vi "Inpterpolate8.vi"(0 "X":fxp<+/-,16,14>, 11 "input valid":bool=TRUE) -> (2 "X(t -7)":fxp<+/-,16,14>, 3 "X(t -5)":fxp<+/-,16,14>, 4 "X(t)":fxp<+/-,16,14>, 6 "X(t -1)":fxp<+/-,16,14>, 8 "X(t -2)":fxp<+/-,16,14>, 10 "X(t -3)":fxp<+/-,16,14>, 13 "X(t -6)":fxp<+/-,16,14>, 14 "X(t -4)":fxp<+/-,16,14>, 15 "output valid":bool)   [LabVIEW 2013]
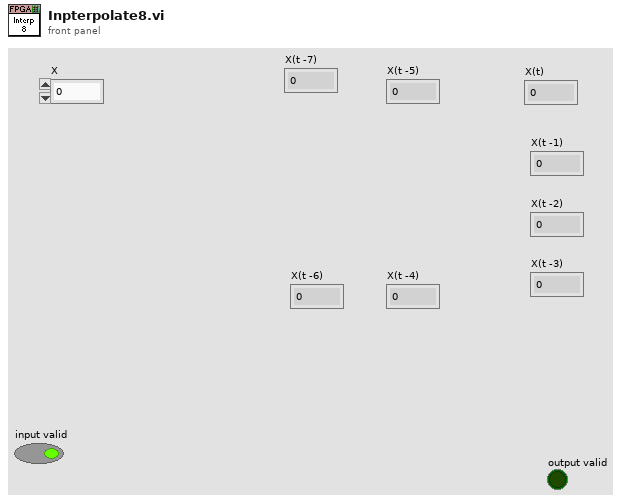
[diagram p1: front panel]
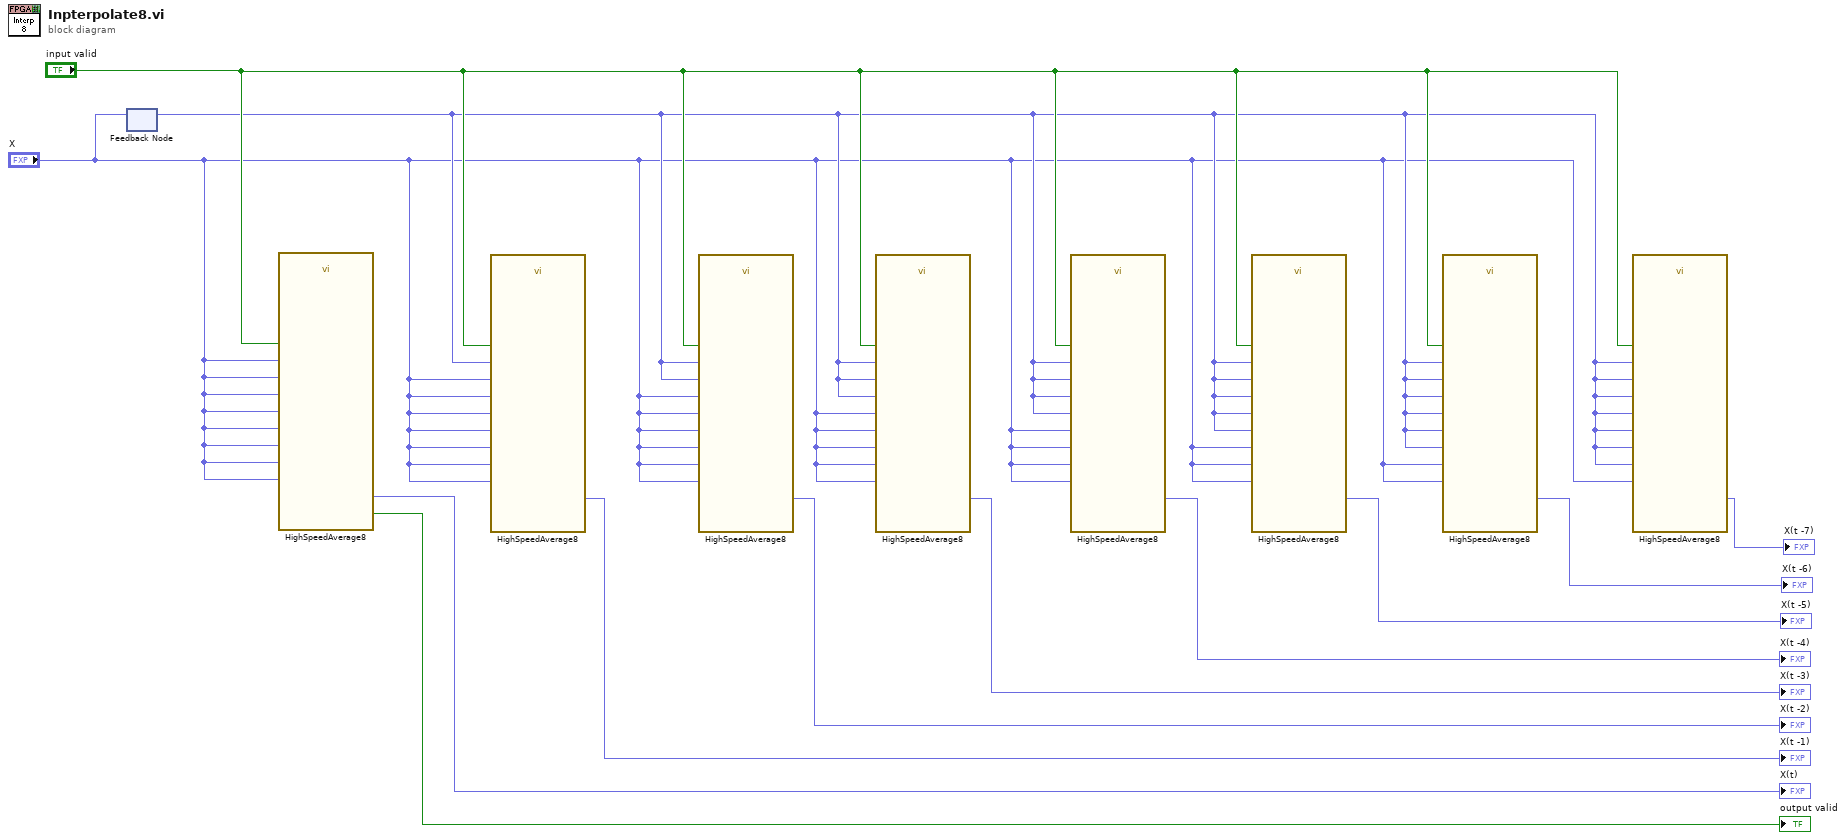
[diagram p0: block diagram]
diagram:
  n1 = feedback #1() -> (w2:fxp<+/-,16,14>)  [unwired: 1 in]
  n2 = feedback-in #1("X") -> ()
  n3 = call "HighSpeedAverage8.vi"("x 1"="X", "x 5"="X", "x 6"="X", "x 2"="X", "x 3"="X", "x 4"="X", "input valid"="input valid", "x 7"="X", "x 8"="X") -> ("average"=→"X(t)":fxp<+/-,16,14>, "output valid"=→"output valid":bool)  [unwired: 5 in]
  n4 = call "HighSpeedAverage8.vi"("x 1"=w2, "x 5"="X", "x 6"="X", "x 2"="X", "x 3"="X", "x 4"="X", "input valid"="input valid", "x 7"="X", "x 8"="X") -> ("average"=→"X(t -1)":fxp<+/-,16,14>)  [unwired: 5 in, 1 out]
  n5 = call "HighSpeedAverage8.vi"("x 1"=w2, "x 5"="X", "x 6"="X", "x 2"=w2, "x 3"="X", "x 4"="X", "input valid"="input valid", "x 7"="X", "x 8"="X") -> ("average"=→"X(t -2)":fxp<+/-,16,14>)  [unwired: 5 in, 1 out]
  n6 = call "HighSpeedAverage8.vi"("x 1"=w2, "x 5"="X", "x 6"="X", "x 2"=w2, "x 3"=w2, "x 4"="X", "input valid"="input valid", "x 7"="X", "x 8"="X") -> ("average"=→"X(t -3)":fxp<+/-,16,14>)  [unwired: 5 in, 1 out]
  n7 = call "HighSpeedAverage8.vi"("x 1"=w2, "x 5"="X", "x 6"="X", "x 2"=w2, "x 3"=w2, "x 4"=w2, "input valid"="input valid", "x 7"="X", "x 8"="X") -> ("average"=→"X(t -4)":fxp<+/-,16,14>)  [unwired: 5 in, 1 out]
  n8 = call "HighSpeedAverage8.vi"("x 1"=w2, "x 5"=w2, "x 6"="X", "x 2"=w2, "x 3"=w2, "x 4"=w2, "input valid"="input valid", "x 7"="X", "x 8"="X") -> ("average"=→"X(t -5)":fxp<+/-,16,14>)  [unwired: 5 in, 1 out]
  n9 = call "HighSpeedAverage8.vi"("x 1"=w2, "x 5"=w2, "x 6"=w2, "x 2"=w2, "x 3"=w2, "x 4"=w2, "input valid"="input valid", "x 7"="X", "x 8"="X") -> ("average"=→"X(t -6)":fxp<+/-,16,14>)  [unwired: 5 in, 1 out]
  n10 = call "HighSpeedAverage8.vi"("x 1"=w2, "x 5"=w2, "x 6"=w2, "x 2"=w2, "x 3"=w2, "x 4"=w2, "input valid"="input valid", "x 7"=w2, "x 8"="X") -> ("average"=→"X(t -7)":fxp<+/-,16,14>)  [unwired: 5 in, 1 out]
